vi "Error Handler.vi"(8 "error in (no error)":errorcluster, 11 "VISA resource name":refnum<visa-resource-name>) -> (0 "error out":errorcluster, 1 "Error Message":string, 3 "VISA resource name out":refnum<visa-resource-name>)   [LabVIEW 2025, in "Detector SCPI.lvlib"]
doc: "Takes error code and responds accordingly"
uses:
  Detector SCPI.lvlib
panel:
  out "Result":i32
  out "Error Code 2":T1(ring)
  # "EDIT: Note: The Error Query VI is included as a subVI in all driver VIs except low-level API VIs. If the instrument does not support error query, then remove the VI and remove subVI calls in each instrument driver VI that calls it."
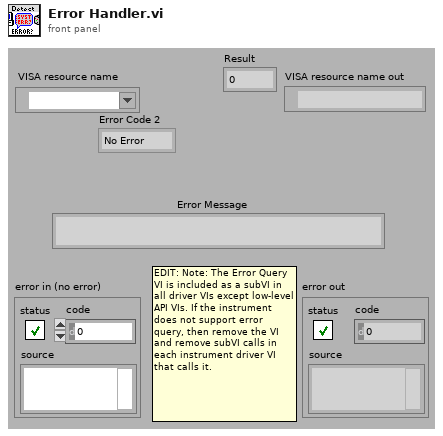
[diagram p1: front panel]
types:
  T1 = enum16{"No Error", "Bad Command", "TImeout", "Buffer Overflow", "Bad Suffix", "Bad Parameter"}
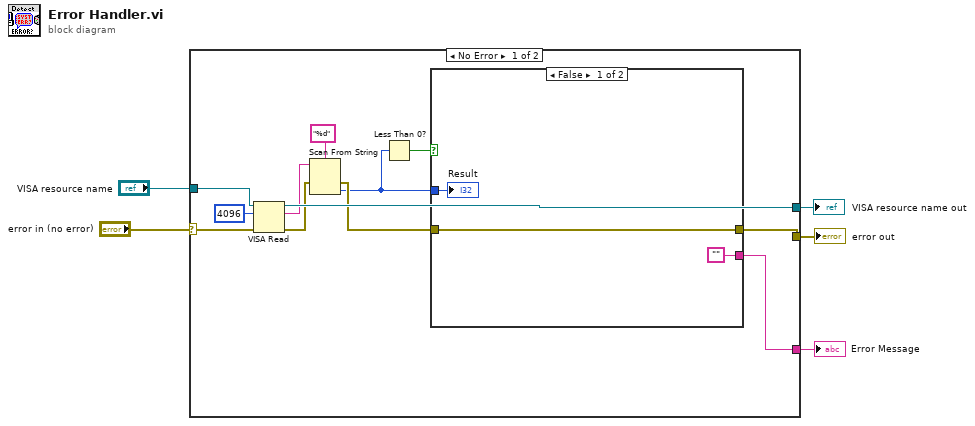
[diagram p0: block diagram]
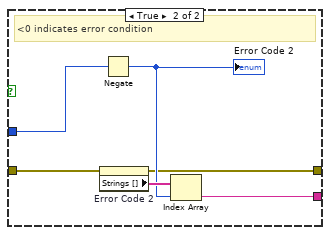
[diagram p2: hidden frame]
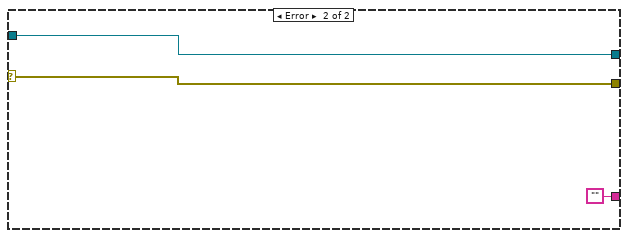
[diagram p3: hidden frame]
diagram:
  n1 = case shown="No Error" "error in (no error)" {
    selector: "error in (no error)" -> [w15 w27]
    tunnel: [w13 w29] -> w5
    tunnel: "VISA resource name" -> [w14 w29]
    tunnel: [w17 w27] -> w4
    tunnel: [w16 ""] -> w3
    frame No Error {
      n2 = VISA Read(VISA resource name=w14, byte count=u32 4096, error in (no error)=w15) -> (VISA resource name out=w13:refnum<visa-resource-name>, read buffer=w11:string, error out=w9:errorcluster)  [unwired: 1 out]
      n3 = Scan From String(format string="%d", input string=w11, error in=w9) -> (error out=w8:errorcluster, output 1=w6:i32)  [unwired: 2 in, 2 out]
      n4 = Less Than 0?(x=w6) -> (x < 0?=w7:bool)
      n5 = case shown="False" w7 {
        tunnel: [w20 w24] -> w17
        tunnel: ["" w23] -> w16
        tunnel: w6 -> [w18 w22]
        tunnel: w8 -> [w20 w21]
        frame False {
          "Result" <- w18
        }
        frame True {
          # "<0 indicates error condition"
          n6 = property on="Error Code 2" class="Enum (strict)"(error in=w21) -> (error out=w24:errorcluster, "Strings []"=w26:string[])  [unwired: 1 in, 1 out]
          n7 = Negate(x=w22) -> (-x=w25:i32)
          "Error Code 2" <- w25
          n8 = Index Array(array=w26, index=w25) -> (element=w23:string)
        }
      }
    }
    frame Error {
    }
  }
  "VISA resource name out" <- w5
  "error out" <- w4
  "Error Message" <- w3
